vi "Omron_Monitor_Mode.vi"(8 "error in":errorcluster, 11 "COM in":refnum<visa-resource-name>) -> (0 "error out":errorcluster, 3 "COM out":refnum<visa-resource-name>)   [LabVIEW 2015]
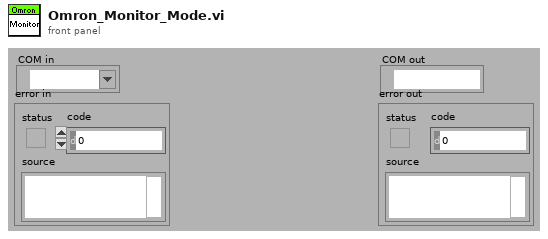
[diagram p1: front panel]
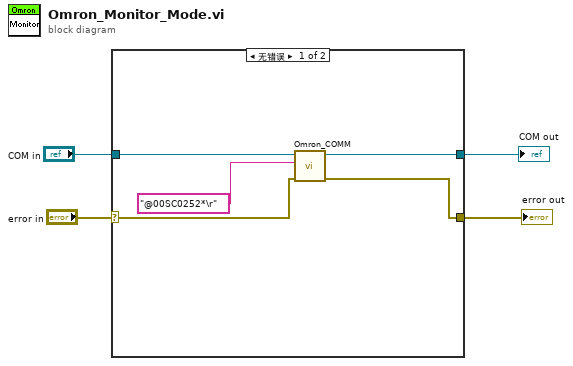
[diagram p0: block diagram]
diagram:
  n1 = case shown="无错误" "error in" {
    selector: "error in" -> [w7 w10]
    tunnel: [w5 w10] -> w4
    tunnel: [w6 w11] -> w3
    tunnel: "COM in" -> [w8 w11]
    frame No Error {
      n2 = call "Omron_COMM.vi"("error in"=w7, "Write data"="@00SC0252*\r" ("write buffer"), "COM in"=w8) -> ("error out"=w5:errorcluster, "COM out"=w6:refnum<visa-resource-name>)  [unwired: 6 in, 1 out]
    }
    frame Error {
    }
  }
  "error out" <- w4
  "COM out" <- w3
